vi "amc_Get Local Name and IP.vi"(11 "Reset":bool) -> (1 "IP Address":string, 2 "Short Name":string, 3 "Name":string)   [LabVIEW 2017]
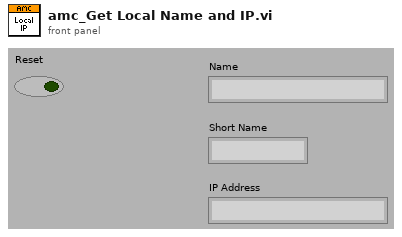
[diagram p1: front panel]
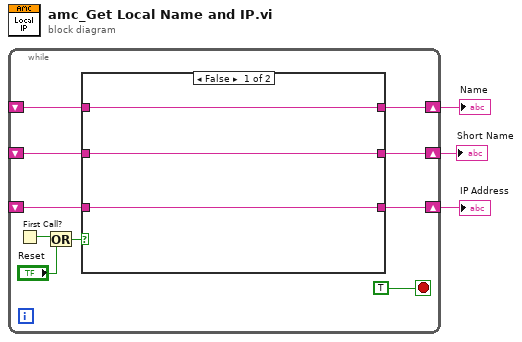
[diagram p0: block diagram]
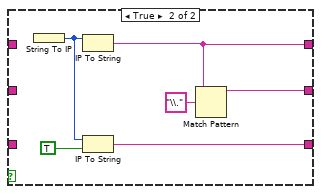
[diagram p2: hidden frame]
diagram:
  n1 = while {
    shift-right: [w8] -> w3
    shift-left: _ -> [w6]
    shift-right: [w9] -> w2
    shift-left: _ -> [w5]
    shift-right: [w7] -> w1
    shift-left: _ -> [w4]
    stop <- TRUE stop-if-true
    n2 = First Call?() -> (First Call?: T/F=w12:bool)
    n3 = Or(x=w12, y="Reset") -> (x .or. y?=w10:bool)
    n4 = case shown="False" w10 {
      tunnel: [w15 w19] -> w9
      tunnel: [w16 w18] -> w8
      tunnel: [w14 w17] -> w7
      tunnel: w6 -> [w16 _]
      tunnel: w5 -> [w15 _]
      tunnel: w4 -> [w14 _]
      frame False {
      }
      frame True {
        n5 = String To IP() -> (0:w21:u32)  [unwired: 1 out]
        n6 = IP To String(2:w21) -> (0:w18:string)  [unwired: 1 out]
        n7 = IP To String(1:TRUE ("dot notation? (F)"), 2:w21) -> (0:w17:string)
        n8 = Match Pattern(string=w18, regular expression="\\.") -> (before substring=w19:string)  [unwired: 4 out]
      }
    }
  }
  "Name" <- w3
  "Short Name" <- w2
  "IP Address" <- w1
